vi "optionsAcq_spectralRange_waveNr.vi"(0 "reference":refnum<class "OSA300.lvclass">, 1 "range min (waveNr)":sgl, 2 "range max (waveNr)":sgl, 3 "write action":enum16{"range min", "range max", "both"}(ring), 4 "readWrite":enum16{"read", "write"}(ring), 5 "error in (no error)":errorcluster) -> (14 "duplicate reference":refnum<class "OSA300.lvclass">, 15 "range min read (waveNr)":sgl, 16 "range max read (waveNr)":sgl, 19 "error out":errorcluster)   [LabVIEW 2010, in "OSA300.lvclass"]
doc: "optionsAcq_spectralRange_waveNr enables a reduction of the spectrum dataset size while maintaining resolution. This is done by calling the functions 'FTS_SetAcquisitionOption_MinWaveNr' and 'FTS_SetAcquisitionOption_MaxWaveNr' with the desired wavenumber range. \n\nNotice that this cutting is done during the calculation of the spectrum from the interferogram and does not affect the interferogram at all, nor the time required to perform a measurement, (spectra update time unchanged).\n\nA smaller spectrum dataset can also be obtained by switching to low resolution mode. \n\nIn write mode; the spectrum graph x range will be updated accordingly, (plot_spectrum.vi will update graph with new range). This applies to spectrum graph which reference has been wired to init.vi., (see tree.vi for compatible graph).\n\nIn write both mode; the range min and max will be swapped if min being larger than max."
uses:
  OSA300.lvclass
  OSA.lvclass
  OSA300.lvclass/OSA300.ctl
  _OSAchannel_class/OSAchannel.lvclass
  FTSLib.dll
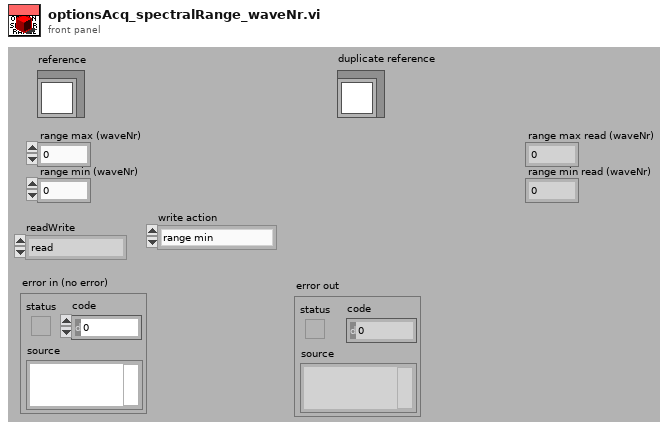
[diagram p1: front panel]
types:
  T1 = typedef "OSA.lvclass/interferogram_smoothing.ctl" = enum16{"NONE", "BINOMIAL", "SAVITSKY_GOLAY", "FOURIER", "MOVING_AVERAGE", "GAUSSIAN"}
  T2 = cluster{"waveMin (cm-1)":sgl, "waveMax (cm-1)":sgl, "gainOffset_auto":bool, "gain":i32, "gain levels nr":u16, "offset":i32, "offset max":u16, "damper available":bool, "damper active":bool, "amplifier type":i32, "detector type":i32, "channelIdx global":u16, "spectrIdx":u16, "waveMeter on":bool, "ref gainLevels rel.":refnum<data-value>, "intfgrm_smooth_width":u16, "intfgrm_smooth_nrOfPasses":u16, "intfgrm_smooth":T1, "adc #bits":dbl, "temp Variable":bool, "spectr_smooth":T1, "spectr_smooth_width":u16, "spectr_smooth_nrOfPasses":u16}
  T3 = typedef "OSA.lvclass/ObjectAttributes.ctl" = cluster{"Stop":bool, "dataType":T4, "spectrometerIdx":u16, "buffer size interferogram":i32, "interferogram":cluster{"new":bool, "plot_x_ min":sgl, "plot_x_max":sgl, "plot_y_min":sgl, "plot_y_max":sgl, "Graph Intrfrgrm":T5, "timeStamp":u32, "signal (%)":dbl, "traces":cluster{"idx":u32, "broadBand":bool, "monoChromatic":bool, "peakToPeakSignal":dbl, "peakToPeakPos":dbl}[], "traces idx last":i32}, "spectrum":cluster{"new":bool, "plot_x_min":sgl, "plot_x_max":sgl, "plot_unit_x":T6, "plot_unit_y":T7, "plot_y_min":sgl, "plot_y_max":sgl, "Graph Spectrum":T5, "timeStamp":u32, "X_VAL_OPTIONS":enum16{"MIN_MAX", "ARRAY"}, "traces":cluster{"idx":u32}[], "traces idx last":i32}, "Thorlabs_OSA_64.lvclass:queue_action.ctlqueue ref":refnum<queue>, "action":T8, "plot zoom step":dbl, "buffer semaphore":T9, "acq stopped":bool, "dataType active":T4, "temperature (degr C)":sgl, "pressure (hPa)":sgl, "rel humidity (%)":sgl, "settings":cluster{"resolution":T10, "sensitivity":T11, "Average":bool, "average nr":u32, "apodisation":T12, "acq delay (ms)":u32, "airMesure":T13, "wmtr on":bool, "intfgrm_smooth_width":u16, "intfgrm_smooth_nrOfPasses":u16, "intfgrm_smooth":T1, "phaseCorrection":T14, "zeroFill":u8, "spectr_smooth":T1, "spectr_smooth_width":u16, "spectr_smooth_nrOfPasses":u16, "resolution (/cm)":sgl, "REF wavelength, (nm)":dbl, "gain_idx":u16, "gainAuto":bool, "gain_relative":dbl, "PD sensitivity mode":T15, "PD senseMode implemented":bool, "SensorTemperature implemented":bool, "SensorPressure implemented":bool, "SensorHumidity implemented":bool}, "peaks position":sgl[], "peaks width":sgl[], "peaks height":sgl[], "peaks max nr":u32, "peaks latest nr":i32, "peaks new":bool, "power":dbl, "power new":bool, "path":string, "wavelength (WNr)":dbl, "wavelength new":bool, "buffer size spectrum":i32, "status":string, "VI reference":refnum<vi>, "funcPointer":u64, "libraryPointer":u64, "singleAcquisition":bool, "coherenceLength (cm)":dbl, "coherenceLength new":bool, "spectrometer model":string, "spectrometer serial nr":string, "peaks thld left":sgl[], "peaks thld right":sgl[], "coherenceLength error (cm)":dbl, "ADC bits":u16, "peaks position centroid":sgl[], "peaks height centroid":sgl[], "OSA series":T16, "channel index spectrum":u16, "spectrometer rangeLow, (/cm)":dbl, "spectrometer rangeHigh, (/cm)":dbl, "channel index interferogram":u16}
  T4 = typedef "OSA.lvclass/acq_dataType.ctl" = enum16{"none", "interferogram", "spectrum"}
  T5 = typedef "OSA.lvclass/graph_intensity.ctl" = refnum<vi>
  T6 = typedef "OSA.lvclass/spectrum_x_unit.ctl" = enum16{"wavenr/cm", "THz", "eV", "nm_air", "nm_vac"}
  T7 = typedef "OSA.lvclass/y_unit.ctl" = enum16{"ADC counts", "dBm pwr absolute", "dBm pwr density", "mW pwr absolute", "mW pwr density"}
  T8 = typedef "OSA.lvclass/queue_action.ctl" = enum16{"none", "stop", "GUI_plotInterferogram", "GUI_plotSpectrum", "GUI_plotInterferogramRescale", "GUI_plotSpectrumRescale", "GUI_plotInterferogramReset", "GUI_plotSpectrumReset", "GUI_plotInterferogramAutoScaleY", "GUI_plotSpectrumAutoScaleY", "GUI_plotInterferogramZoomOut", "GUI_plotSpectrumZoomOut", "GUI_plotInterferogramPane", "GUI_plotSpectrumPane", "GUI_plotInterferogramZoomMouse", "GUI_plotSpectrumZoomMouse", "ENVIRONMENT temperature", "ENVIRONMENT pressure", "MODE_resolution set", "MODE_resolution get", "MODE_sensitivity set", "MODE_sensitivity get", "MODE_PDTemperature set", "MODE_PDTemperature get", "REBOOT/RESET firmware", "ACQASYNC_acquireSingleSpectrum", "ACQASYNC_continuous start", "ACQASYNC_continuous stop\n", "ACQASYNC_get last interferogram", "ACQASYNC_get last spectrum", "ACQASYNC_get last waveNr", "ACQOPT_interferogram smoothing set", "ACQOPT_interferogram smoothing get", "ACQOPT_spectrum smoothing set", "ACQOPT_spectrum smoothing get", "ACQOPT_apodisation type set", "ACQOPT_apodisation type get", "ACQOPT_phase correction type set", "ACQOPT_phase correction type get", "ACQOPT_acqIntervall_set", "ACQOPT_acqIntervall_get", "ACQOPT_average spectrum set", "ACQOPT_average spectrum get", "ACQOPT_rolling average set", "ACQOPT_rolling average get", "ACQOPT_zero fill factor set", "ACQOPT_zero fill factor get", "ACQOPT_cycle counting set", "ACQOPT_cycle counting get", "ACQOPT_air measure option set", "ACQOPT_air measure option get", "ACQOPT_gainLevel auto get", "ACQOPT_gainLevel auto set", "ACQOPT_gainLevel get", "ACQOPT_gainLevel set", "ACQOPT_getAll", "INSTRUMENT_PROPERTY_range_WaveNr_min", "INSTRUMENT_PROPERTY_range_WaveNr_max", "INSTRUMENT_PROPERTY_reference_wavelength_cm^-1", "INSTRUMENT_PROPERTY_samplesPerRefPeriod", "INSTRUMENT_PROPERTY_resolution_waveNrPercm", "INSTRUMENT_PROPERTY_availableGainLevels", "INSTRUMENT_PROPERTY_status", "CONVERT", "ANALYSE_POWER", "ANALYSE_PEAKS", "ANALYSE_WAVELENGTH", "ANALYSE_SPECTRUM", "ANALYSE_INTERFEROGRAM", "ANALYSE_COHERENCE_LENGTH", "MATH", "MATH_power", "MATH_peaks", "FILE", "miscellaneous"}
  T9 = typedef "Semaphore RefNum" = refnum<k1>
  T10 = typedef "OSA.lvclass/resolution.ctl" = enum16{"low", "high"}
  T11 = typedef "OSA.lvclass/sensitivityMode.ctl" = enum16{"low", "low medium", "high medium", "high"}
  T12 = typedef "OSA.lvclass/apodisation.ctl" = enum16{"NONE", "NORTON_BEER_WEAK", "NORTON_BEER_MEDIUM", "NORTON_BEER_STRONG", "TRIANGULAR", "COSINE", "HANN", "HAMMING", "BLACKMANHARRIS3", "BLACKMANHARRIS4", "GAUSSIAN"}
  T13 = typedef "OSA.lvclass/airMeasure.ctl" = enum16{"TEMPERATURE", "PRESSURE"}
  T14 = typedef "OSA.lvclass/phaseCorrection.ctl" = enum16{"NONE", "MERTZ", "FORMAN", "MERTZ_FILE", "FORMAN_FILE", "FUTURE COMP."}
  T15 = typedef "OSA.lvclass/PDTemperatureMode.ctl" = enum16{"cool: better sensitivity/noise floor", "warm: extended wl range"}
  T16 = typedef "OSA.lvclass/OSA_series.ctl" = enum16{"OSA200", "OSA300", "UNKNOWN"}
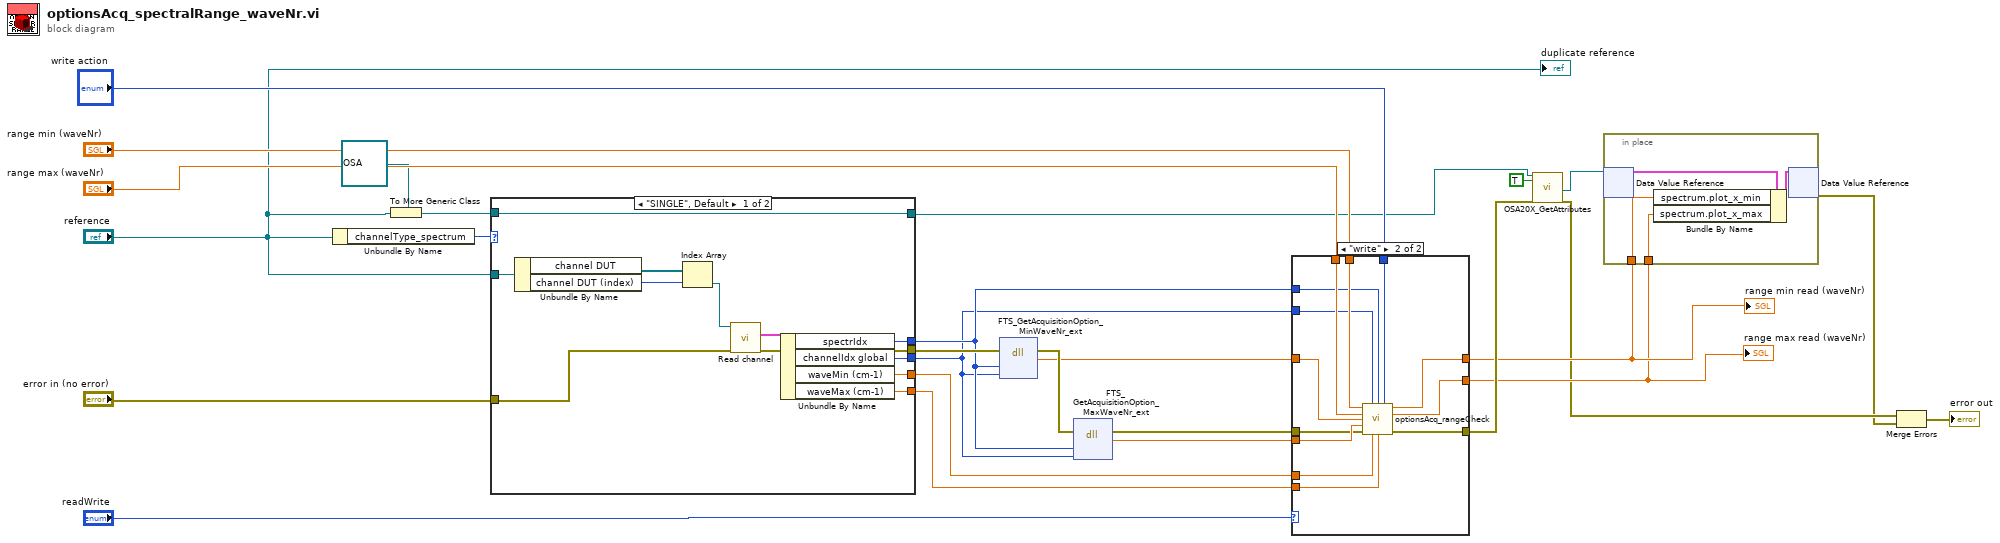
[diagram p0: block diagram]
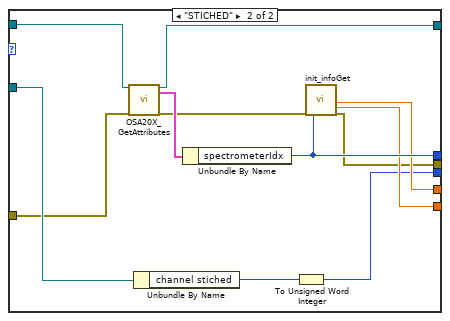
[diagram p2: hidden frame]
diagram:
  n1 = Unbundle By Name("reference") -> ("channelType_spectrum"=w27:enum16{"SINGLE", "STICHED"})
  n2 = To More Generic Class(target class=refnum<class "OSA.lvclass"> refnum ("Thorlabs_OSA_64"), reference="reference") -> (generic class reference=w2:refnum<class "OSA.lvclass">)
  n3 = case shown="\"SINGLE\", Default" w27 {
    tunnel: "reference" -> [w30 w51]
    tunnel: [w35 w43] -> w21
    tunnel: [w34 w45] -> w18
    tunnel: [w33 w44] -> w17
    tunnel: [w32 w46] -> w15
    tunnel: [w31 w42] -> w14
    tunnel: "error in (no error)" -> [w29 w50]
    tunnel: w2 -> [w28 w41]
    tunnel: [w28 w40] -> w1
    frame "SINGLE", Default {
      n4 = Unbundle By Name(w30) -> ("channel DUT"=w39:refnum<class "OSAchannel.lvclass">[], "channel DUT (index)"=w38:i32)
      n5 = Index Array(array=w39, index=w38) -> (element=w37:refnum<class "OSAchannel.lvclass">)
      n6 = call "Read channel.vi"("error in (no error)"=w29, "OSAchannel in"=w37) -> ("error out"=w35:errorcluster, "channel"=w36:T2)  [unwired: 7 in, 1 out]
      n7 = Unbundle By Name(w36) -> ("spectrIdx"=w32:u16, "channelIdx global"=w31:u16, "waveMin (cm-1)"=w34:sgl, "waveMax (cm-1)"=w33:sgl)
    }
    frame "STICHED" {
      n8 = call "OSA20X_GetAttributes.vi"("reference in"=w41, "error in (no error)"=w50) -> ("reference out"=w40:refnum<class "OSA.lvclass">, "Data"=w49:T3, "error out"=w47:errorcluster)  [unwired: 14 in, 1 out]
      n9 = Unbundle By Name(w51) -> ("channel stiched"=w48:u32)
      n10 = Unbundle By Name(w49) -> ("spectrometerIdx"=w46:u16)
      n11 = To Unsigned Word Integer(number=w48) -> (unsigned 16bit integer=w42:u16)
      n12 = call "init_infoGet.vi"("error in (no error)"=w47, "spectrIdx"=w46) -> ("waveNrMin"=w45:sgl, "waveNrMax"=w44:sgl, "error out"=w43:errorcluster)  [unwired: 14 in, 1 out]
    }
  }
  n13 = dll-call lib="FTSLib.dll" fn="FTS_GetAcquisitionOption_MinWaveNr_ext" label="FTS_GetAcquisitionOption_MinWaveNr"(error in=w21, "spectrIdx"=w15, "channel"=w14) -> (error out=w22:errorcluster, "return type"=w20:sgl)  [unwired: 4 in, 1 out]
  n14 = dll-call lib="FTSLib.dll" fn="FTS_GetAcquisitionOption_MaxWaveNr_ext" label="FTS_GetAcquisitionOption_MaxWaveNr"(error in=w22, "spectrIdx"=w15, "channel"=w14) -> (error out=w16:errorcluster, "return type"=w19:sgl)  [unwired: 4 in, 1 out]
  n15 = case shown="\"write\"" "readWrite" {
    tunnel: w20 -> [w54 w67]
    tunnel: w19 -> [w53 w66]
    tunnel: w18 -> [_ w65]
    tunnel: w17 -> [_ w64]
    tunnel: "range min (waveNr)" -> [_ w63]
    tunnel: "range max (waveNr)" -> [_ w62]
    tunnel: w16 -> [w52 w61]
    tunnel: "write action" -> [_ w60]
    tunnel: w15 -> [_ w59]
    tunnel: w14 -> [_ w58]
    tunnel: [w54 w57] -> w9
    tunnel: [w53 w56] -> w8
    tunnel: [w52 w55] -> w12
    frame "read", Default {
    }
    frame "write" {
      n16 = call "optionsAcq_rangeCheck.vi"("range min (waveNr)"=w63, "channel index spectrum"=w58, "spectrometerIdx"=w59, "update mode"=w60, "range max (waveNr)"=w62, "range current min"=w67, "range current max"=w66, "error in"=w61, "waveNrMin support"=w65, "waveNrMax support"=w64) -> ("range min (waveNr) out"=w57:sgl, "range max (waveNr) out"=w56:sgl, "error out"=w55:errorcluster)  [unwired: 3 in]
    }
  }
  "range max read (waveNr)" <- w8
  "range min read (waveNr)" <- w9
  n17 = call "OSA20X_GetAttributes.vi"("reference in"=w1, "OnlyGetDvrReference(False)"=TRUE, "error in (no error)"=w12) -> ("DataRef"=w10:refnum<data-value>, "error out"=w7:errorcluster)  [unwired: 13 in, 2 out]
  n18 = in-place {
    in-place-border: w9 -> [w70]
    in-place-border: w8 -> [w69]
    n19 = in-place-dvr #1(w10) -> (w71:T3)  [unwired: 1 out]
    n20 = Bundle By Name(cluster=w71, "spectrum.plot_x_min"=w70, "spectrum.plot_x_max"=w69) -> (w68:T3)
    n21 = in-place-dvr #1(w68) -> (w6:errorcluster)  [unwired: 1 out]
  }
  n22 = Merge Errors(w7, w6) -> (→"error out":errorcluster)
  "duplicate reference" <- "reference"
